vi "top-level app.vi"() -> ()   [LabVIEW 2015]
panel:
  in  "Close":bool
  in  "header":bool
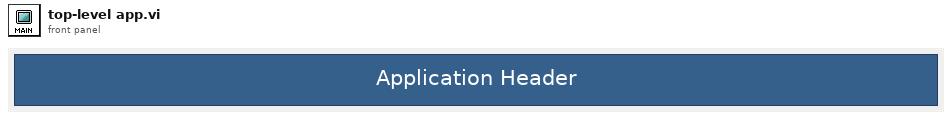
[diagram p1: front panel]
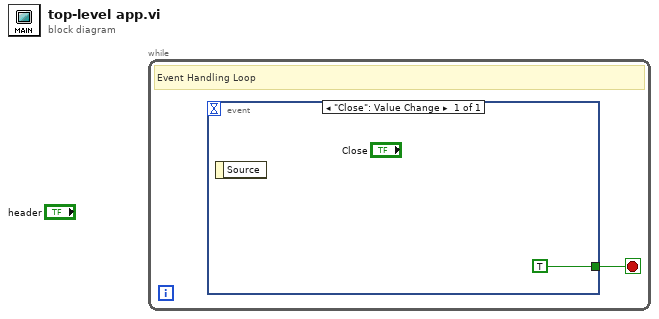
[diagram p0: block diagram]
diagram:
  n1 = while {
    stop <- w1 stop-if-true
    # "Event Handling Loop"
    n2 = event shown="[0] \"Close\": Value Change" {
      selector: _ -> [_]
      dyn-events: _ -> [_]
      timeout: _ -> [_]
      tunnel: [TRUE] -> w1
      event "Close": Value Change {
        n3 = event-data() -> ()  [unwired: 1 in, 1 out]
      }
    }
  }
